vi "Pockels Cal-Modify cursor indexes in file.vi"(7 "Function":enum16{"Whole cal", "Cursors section"}(ring), 9 "SINGLE CAL SET / Pockels Cal table":string[][](array[string]), 10 "Cal files listbox":refnum<vi>, 11 "XYGraph in":refnum<vi>) -> (3 "All data loaded":string[][](array[string]))   [LabVIEW 2013]
uses:
  <vilib>/Utility/error.llb/DialogType.ctl
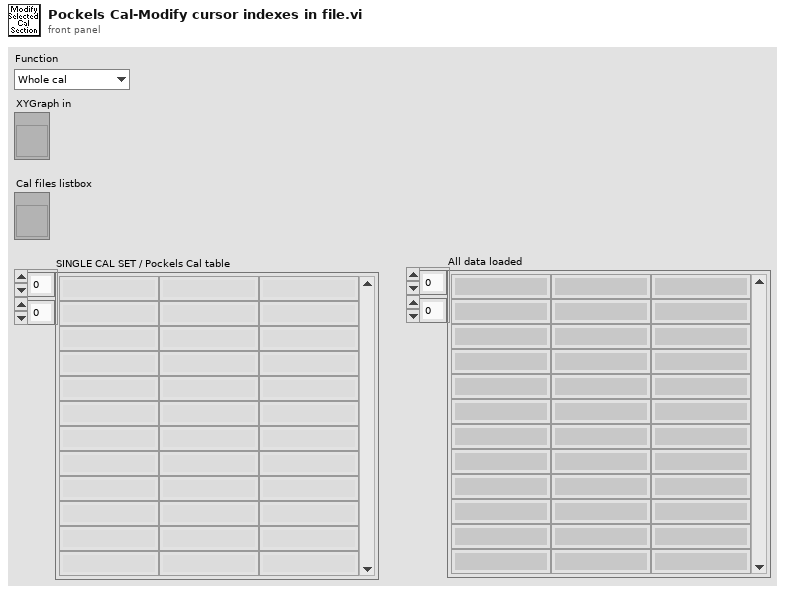
[diagram p1: front panel]
types:
  T1 = typedef "DialogType.ctl" = u16
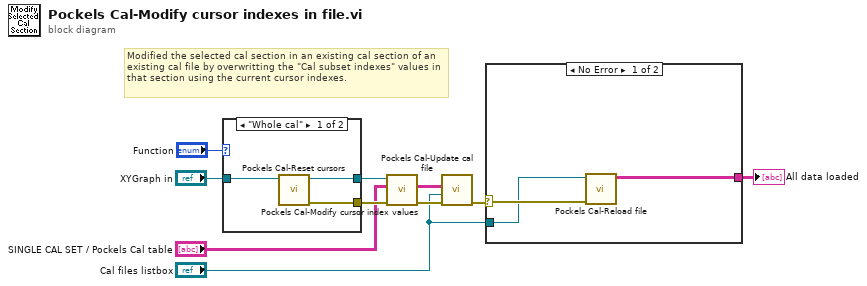
[diagram p0: block diagram]
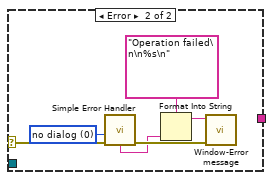
[diagram p2: hidden frame]
diagram:
  # "Modified the selected cal section in an existing cal section of an existing cal file by overwritting the \"Cal subset indexes\" values in that section using the current cursor indexes."
  n1 = case shown="\"Whole cal\"" "Function" {
    tunnel: [w13 _] -> w10
    tunnel: [w12 w14] -> w9
    tunnel: "XYGraph in" -> [w11 w14]
    frame "Whole cal" {
      n2 = call "Pockels Cal-Reset cursors.vi"("XYGraph in"=w11) -> ("error out"=w13:errorcluster, "XYGraph"=w12:refnum<vi>)  [unwired: 9 in]
    }
    frame "Cursors section", Default {
    }
  }
  n3 = call "Pockels Cal-Modify cursor index values.vi"("error in (no error)"=w10, "Single Cal table (Final format)"="SINGLE CAL SET / Pockels Cal table", "XYGraph in"=w9) -> ("error out"=w4:errorcluster, "Single Cal table (Final format)"=w8:string[][])  [unwired: 6 in, 1 out]
  n4 = call "Pockels Cal-Update cal file.vi"("error in (no error)"=w4, "Cal files listbox"="Cal files listbox", "New cal section"=w8) -> ("error out"=w3:errorcluster)  [unwired: 8 in]
  n5 = case shown="No Error" w3 {
    selector: w3 -> [w17 w23]
    tunnel: "Cal files listbox" -> [w16 _]
    tunnel: [w15 _] -> w1
    frame No Error {
      n6 = call "Pockels Cal-Reload file.vi"("error in (no error)"=w17, "Cal files listbox"=w16) -> ("All data loaded"=w15:string[][])  [unwired: 8 in, 1 out]
    }
    frame Error {
      w22 = T1 0 items=["no dialog", "OK message", "continue or stop message", "OK message + warnings", "continue/stop + warnings"] ("type of dialog (OK msg:1)")
      n7 = call <vilib>:"Simple Error Handler.vi"("type of dialog (OK msg:1)"=w22, "error in (no error)"=w23) -> ("error out"=w21:errorcluster, "message"=w19:string)  [unwired: 3 in, 3 out]
      n8 = Format Into String(format string="Operation failed\n\n%s\n", w19) -> (resulting string=w18:string)  [unwired: 2 in, 1 out]
      n9 = call "Window-Error message.vi"("error in (no error)"=w21, "Message"=w18) -> ()  [unwired: 9 in, 1 out]
    }
  }
  "All data loaded" <- w1
